vi "_goop4.llb_Interface_FindInterfaceImplementationVI.vi"(8 "error in (no error)":errorcluster, 10 "Path":path, 11 "LabVIEW Object in":refnum<class>) -> (0 "error out":errorcluster, 2 "VI Refnum Of Interface method in class":refnum<vi>, 3 "NoImplementationFound":bool, 5 "Full Class Name":string)   [LabVIEW 2014]
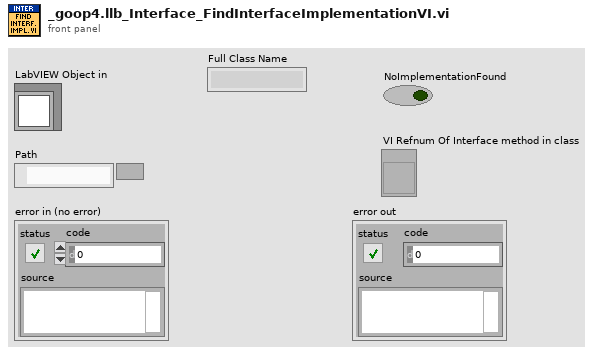
[diagram p1: front panel]
types:
  T1 = enum8{"Only include commented out diagrams if diagram already loaded", "Never include commented out diagrams", "Always include commented out diagrams"}
  T2 = enum8{"No dynamic dispatch VIs", "Include nearest implementation", "Include all overrides"}
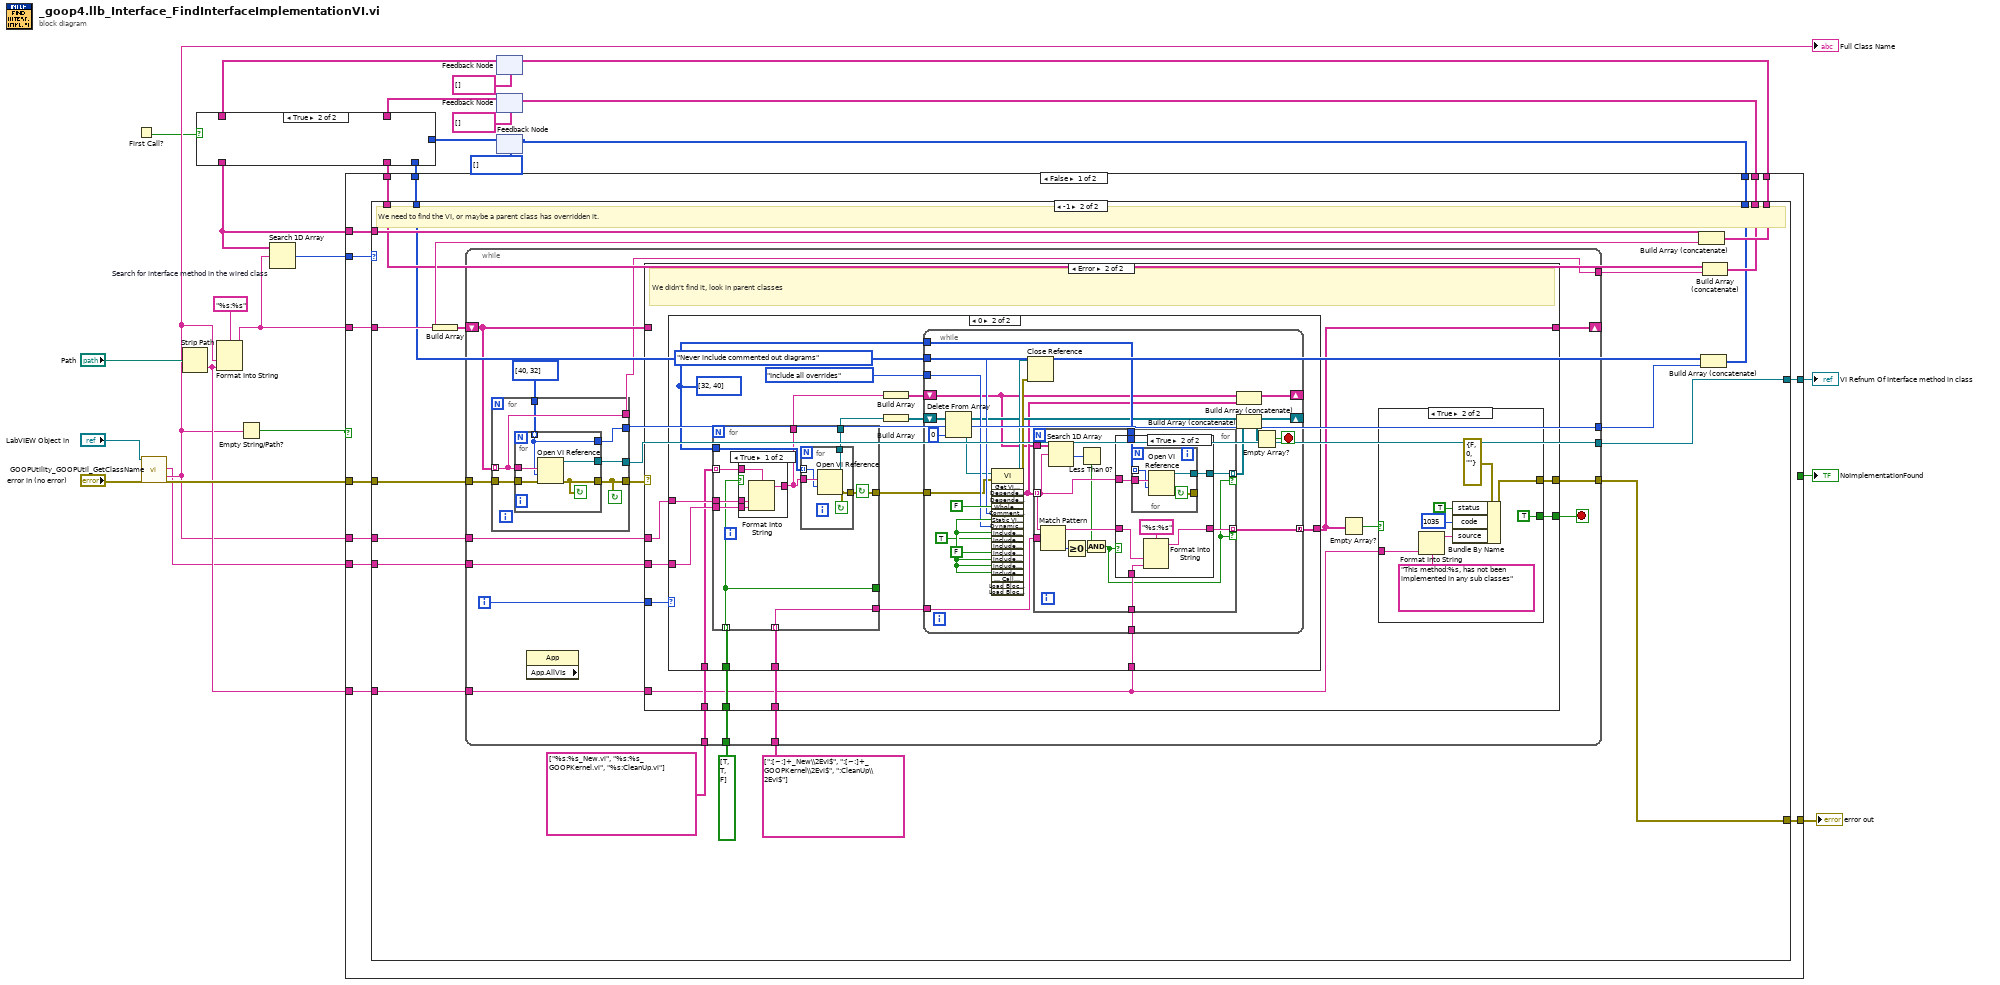
[diagram p0: block diagram]
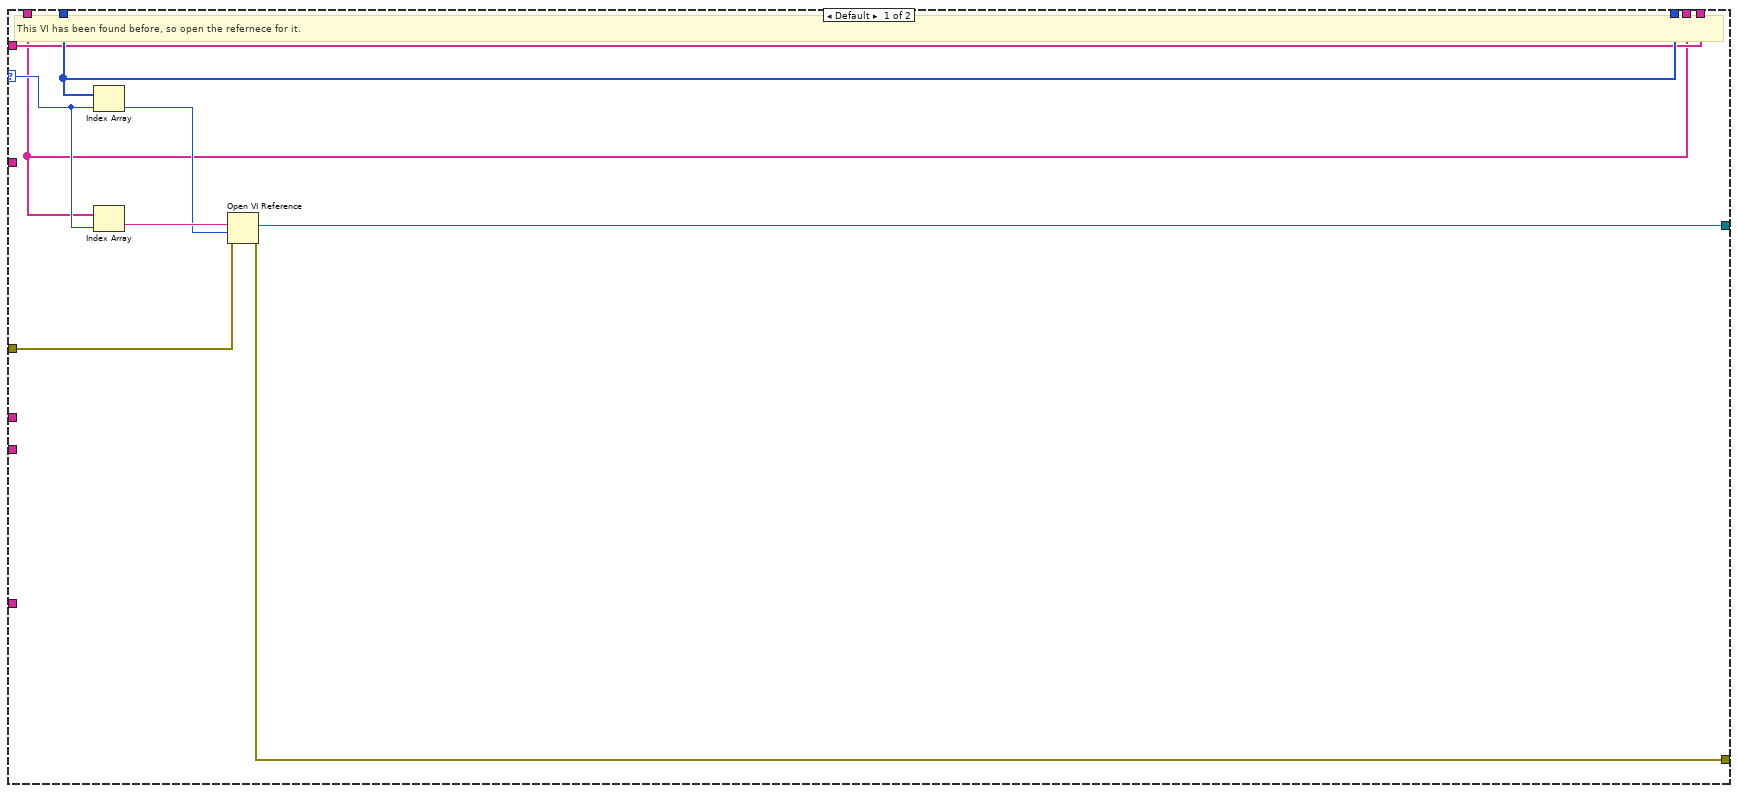
[diagram p2: hidden frame]
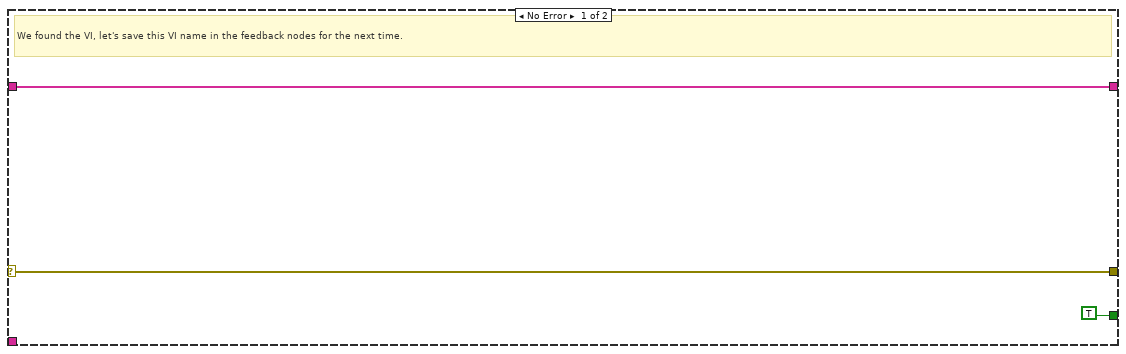
[diagram p3: hidden frame]
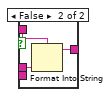
[diagram p6: hidden frame]
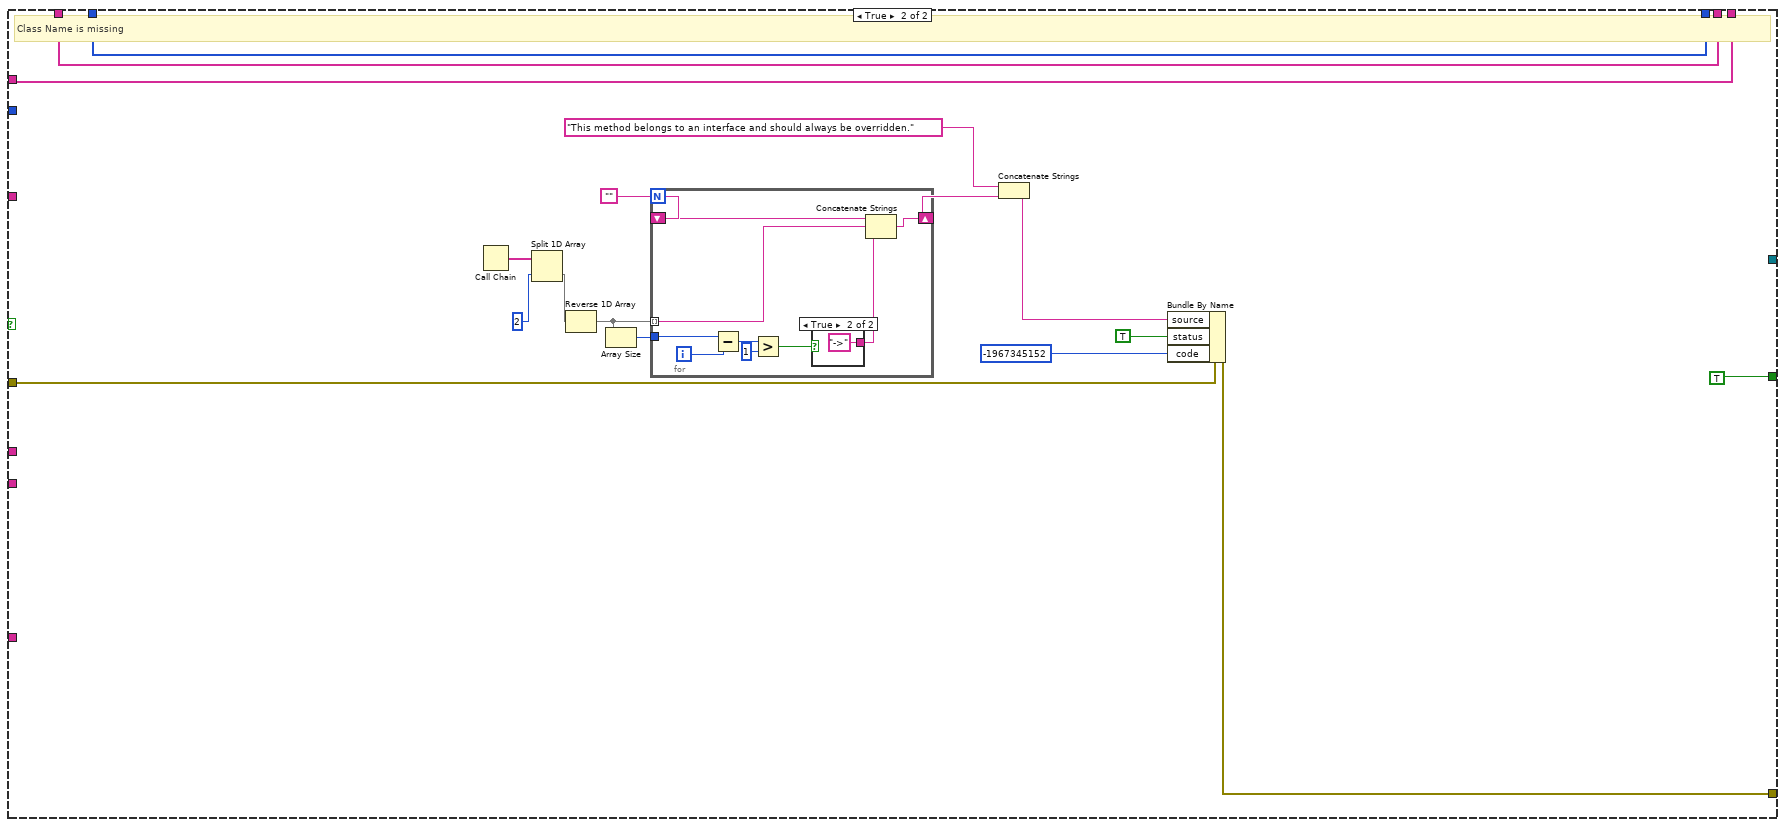
[diagram p8: hidden frame]
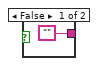
[diagram p9: hidden frame]
diagram:
  n1 = First Call?() -> (First Call?: T/F=w6:bool)
  n2 = call "GOOPUtility_GOOPUtil_GetClassName.vi"("LabVIEW Object"="LabVIEW Object in", "error in (no error)"="error in (no error)") -> ("Class Name"=w10:string, "Full Class Name"=w11:string, "error out"=w22:errorcluster)  [unwired: 13 in, 2 out]
  "Full Class Name" <- w11
  n3 = Strip Path(path="Path") -> (name=w12:string)  [unwired: 1 out]
  n4 = Format Into String(format string="%s:%s", w11, w12) -> (resulting string=w20:string)  [unwired: 2 in, 1 out]
  n5 = Empty String/Path?(string/path=w11) -> (empty?=w2:bool)
  n6 = feedback #1(string[] []) -> (w7:string[])
  n7 = feedback #2(string[] []) -> (w8:string[])
  n8 = feedback #3(i32[] []) -> (w9:i32[])
  n9 = case shown="True" w6 {
    tunnel: w9 -> [w28 _]
    tunnel: w8 -> [w29 _]
    tunnel: w7 -> [w30 _]
    tunnel: [w30 _] -> w5
    tunnel: [w29 _] -> w4
    tunnel: [w28 _] -> w3
    frame False {
    }
    frame True {
    }
  }
  n10 = Search 1D Array "Search for interface method in the wired class"(1D array=w5, element=w20) -> (index of element=w19:i32)  [unwired: 1 in]
  n11 = case shown="False" w2 {
    tunnel: [w44 _] -> w23
    tunnel: w22 -> [w43 w206]
    tunnel: [w42 w205] -> w21
    tunnel: w20 -> [w41 _]
    tunnel: w19 -> [w40 _]
    tunnel: [w39 w219] -> w16
    tunnel: [w38 w221] -> w15
    tunnel: [w37 w220] -> w13
    tunnel: w12 -> [w36 _]
    tunnel: w11 -> [w35 _]
    tunnel: w10 -> [w34 _]
    tunnel: w5 -> [w33 w221]
    tunnel: w4 -> [w32 w220]
    tunnel: w3 -> [w31 w219]
    tunnel: [_ TRUE] -> w1
    frame False {
      n12 = case shown="-1" w40 {
        selector: w40 -> [w51 _]
        tunnel: [w46 w72] -> w44
        tunnel: w43 -> [w48 w71]
        tunnel: [w47 w63] -> w42
        tunnel: w41 -> [_ w68]
        tunnel: w31 -> [w53 w65]
        tunnel: [w53 w64] -> w39
        tunnel: w33 -> [w52 w69]
        tunnel: [w52 w70] -> w38
        tunnel: w32 -> [w45 w67]
        tunnel: [w45 w66] -> w37
        tunnel: w36 -> [_ w62]
        tunnel: w35 -> [_ w58]
        tunnel: w34 -> [_ w57]
        frame Default {
          # "This VI has been found before, so open the refernece for it."
          n13 = Index Array(array=w53, index=w51) -> (element=w49:i32)
          n14 = Index Array(array=w45, index=w51) -> (element=w50:string)
          n15 = Open VI Reference(vi path=w50, options=w49, error in (no error)=w48) -> (vi reference=w46:refnum<vi>, error out=w47:errorcluster)  [unwired: 3 in]
        }
        frame -1 {
          # "We need to find the VI, or maybe a parent class has overridden it."
          n16 = Build Array(w68) -> (w61:string[])
          n17 = while {
            tunnel: [w82] -> w72
            tunnel: w71 -> [w89]
            shift-right: [w85] -> _
            shift-left: w61 -> [w86]
            tunnel: [w84] -> w63
            tunnel: w62 -> [w83]
            tunnel: [w81] -> w60
            tunnel: [w80] -> w59
            tunnel: w58 -> [w78]
            tunnel: w57 -> [w77]
            tunnel: bool[] [TRUE, TRUE, FALSE] -> [w76]
            tunnel: string[] ["%s:%s_New.vi", "%s:%s_GOOPKernel.vi", "%s:CleanUp.vi"] -> [w75]
            tunnel: string[] [":[~:]+_New\\2Evi$", ":[~:]+_GOOPKernel\\2Evi$", ":CleanUp\\2Evi$"] -> [w74]
            i -> [w79]
            stop <- w87 stop-if-true
            n18 = for {
              tunnel: i32[] [40, 32] -> [w91]
              tunnel: w89 -> [w95]
              tunnel: [w94] -> w88
              tunnel: [w93] -> w82
              tunnel: w86 -> [w92] mode=indexing
              tunnel: [w90] -> w81
              tunnel: [w92] -> w80
              stop <- w94 continue-if-true
              n19 = for {
                tunnel: w92 -> [w99]
                tunnel: [w98] -> w93
                tunnel: w91 -> [w96] mode=indexing
                tunnel: w95 -> [w100]
                tunnel: [w97] -> w94
                tunnel: [w96] -> w90
                stop <- w97 continue-if-true
                n20 = Open VI Reference(vi path=w99, options=w96, error in (no error)=w100) -> (vi reference=w98:refnum<vi>, error out=w97:errorcluster)  [unwired: 3 in]
              }
            }
            n21 = property class="App" props=["App.AllVIs"]() -> ()  [unwired: 2 in, 3 out]
            n22 = case shown="Error" w88 {
              selector: w88 -> [w101 _]
              tunnel: [TRUE w113] -> w87
              tunnel: w86 -> [w102 _]
              tunnel: [w102 w105] -> w85
              tunnel: [w101 w114] -> w84
              tunnel: w83 -> [_ w106]
              tunnel: w79 -> [_ w112]
              tunnel: w78 -> [_ w111]
              tunnel: w77 -> [_ w110]
              tunnel: w76 -> [_ w109]
              tunnel: w75 -> [_ w108]
              tunnel: w74 -> [_ w107]
              frame No Error {
                # "We found the VI, let's save this VI name in the feedback nodes for the next time."
              }
              frame Error {
                # "We didn't find it, look in parent classes"
                n23 = case shown="0" w112 {
                  tunnel: w111 -> [_ w130]
                  tunnel: w110 -> [_ w129]
                  tunnel: w109 -> [_ w128]
                  tunnel: w108 -> [_ w127]
                  tunnel: w107 -> [_ w126]
                  tunnel: w106 -> [_ w122]
                  tunnel: [_ w120] -> w105
                  frame Default {
                  }
                  frame 0 {
                    w115 = i32[] [32, 40]
                    n24 = for {
                      tunnel: [w181] -> w118
                      tunnel: [w180] -> w123
                      tunnel: w130 -> [w185]
                      tunnel: w127 -> [w184] mode=indexing
                      tunnel: w128 -> [w178] mode=indexing
                      tunnel: w129 -> [w183]
                      tunnel: [w182] -> w121
                      tunnel: w126 -> [w182] mode=indexing
                      tunnel: w115 -> [w179]
                      tunnel: [w178] -> _
                      tunnel: [w177] -> w116
                      stop <- w180 continue-if-true
                      n25 = case shown="True" w178 {
                        tunnel: [w193 w196] -> w177
                        tunnel: w185 -> [w192 w195]
                        tunnel: w184 -> [w191 w194]
                        tunnel: w183 -> [w190 _]
                        frame True {
                          n26 = Format Into String(format string=w191, w192, w190) -> (resulting string=w193:string)  [unwired: 2 in, 1 out]
                        }
                        frame False {
                          n27 = Format Into String(format string=w194, w195) -> (resulting string=w196:string)  [unwired: 2 in, 1 out]
                        }
                      }
                      n28 = for {
                        tunnel: w177 -> [w189]
                        tunnel: [w188] -> w181
                        tunnel: w179 -> [w187] mode=indexing
                        tunnel: [w186] -> w180
                        stop <- w186 continue-if-true
                        n29 = Open VI Reference(vi path=w189, options=w187) -> (vi reference=w188:refnum<vi>, error out=w186:errorcluster)  [unwired: 4 in]
                      }
                    }
                    n30 = Build Array(w116) -> (w117:string[])
                    n31 = Build Array(w118) -> (w119:refnum<vi>[])
                    n32 = while {
                      tunnel: T2."Include all overrides" ("Dynamic Dispatching?") -> [w143]
                      tunnel: T1."Never include commented out diagrams" ("Commented Out Diagrams?") -> [w144]
                      tunnel: w123 -> [w141]
                      tunnel: w122 -> [w148]
                      tunnel: w121 -> [w147]
                      tunnel: [w146] -> w120 mode=concatenating
                      shift-right: [w135] -> _
                      shift-left: w119 -> [w140]
                      tunnel: w115 -> [w138]
                      shift-right: [w131] -> _
                      shift-left: w117 -> [w132]
                      stop <- w134 stop-if-true
                      w152 = FALSE ("Include Poly VIs?")
                      n33 = Delete From Array(array=w140, index=0) -> (deleted portion=w142:refnum<vi>, array with subset deleted=w136:refnum<vi>[])  [unwired: 1 in]
                      n34 = invoke class="VI" method="Get VI Dependencies"(reference=w142, error in=w141, "Whole Hierarchy?"=FALSE, "Commented Out?"=w144, "Static VI Refs?"=w152, "Dynamic Dispatching?"=w143, "Include Missing VIs?"=w152, "Include Standard VIs?"=TRUE, "Include Poly VIs?"=w152, "Include Global VIs?"=w152, "Include Control VIs?"=w152, "Include Generic VIs?"=w152) -> (reference out=w149:refnum<vi>, error out=w150:errorcluster, "Dependency Names"=w133:string[])  [unwired: 7 in, 16 out]
                      n35 = Close Reference(reference=w149, error in (no error)=w150) -> ()  [unwired: 1 out]
                      n36 = for {
                        tunnel: w147 -> [w161]
                        tunnel: w133 -> [w157] mode=indexing
                        tunnel: [w162] -> w146 mode=indexing if=w153
                        tunnel: w148 -> [w163]
                        tunnel: w138 -> [w160]
                        tunnel: [w159] -> w137 mode=indexing if=w153
                        tunnel: w132 -> [w158]
                        n37 = Match Pattern(string=w157, regular expression=w161) -> (before substring=w164:string, offset past match=w165:i32)  [unwired: 1 in, 2 out]
                        n38 = Search 1D Array(1D array=w158, element=w157) -> (index of element=w156:i32)  [unwired: 1 in]
                        n39 = Greater Or Equal To 0?(x=w165) -> (x >= 0?=w155:bool)
                        n40 = Less Than 0?(x=w156) -> (x < 0?=w154:bool)
                        n41 = And(x=w154, y=w155) -> (x .and. y?=w153:bool)
                        n42 = case shown="True" w153 {
                          tunnel: w164 -> [_ w171]
                          tunnel: w163 -> [_ w170]
                          tunnel: [_ w169] -> w162
                          tunnel: w157 -> [_ w168]
                          tunnel: w160 -> [_ w167]
                          tunnel: [_ w166] -> w159
                          frame False {
                          }
                          frame True {
                            n43 = for {
                              tunnel: w168 -> [w176]
                              tunnel: [w175] -> w166
                              tunnel: w167 -> [w174] mode=indexing
                              tunnel: [w173] -> _
                              stop <- w173 continue-if-true
                              n44 = Open VI Reference(vi path=w176, options=w174) -> (vi reference=w175:refnum<vi>, error out=w173:errorcluster)  [unwired: 4 in]
                            }
                            n45 = Format Into String(format string="%s:%s", w171, w170) -> (resulting string=w169:string)  [unwired: 2 in, 1 out]
                          }
                        }
                      }
                      n46 = Build Array (concatenate)(w132, w133) -> (w131:string[])
                      n47 = Build Array (concatenate)(w136, w137) -> (w135:refnum<vi>[])
                      n48 = Empty Array?(array=w135) -> (empty?=w134:bool)
                    }
                  }
                }
                n49 = Empty Array?(array=w105) -> (empty?=w104:bool)
                n50 = case shown="True" w104 {
                  tunnel: [_ w204] -> w114
                  tunnel: [_ TRUE] -> w113
                  tunnel: w106 -> [_ w200]
                  frame False {
                  }
                  frame True {
                    n51 = Format Into String(format string="This method:%s, has not been implemented in any sub classes" ("string"), w200) -> (resulting string=w201:string)  [unwired: 2 in, 1 out]
                    n52 = Bundle By Name(cluster=errorcluster {"status"=FALSE, "code"=0, "source"=""} ("error IO"), "status"=TRUE, "code"=1035, "source"=w201) -> (w204:errorcluster)
                  }
                }
              }
            }
          }
          n53 = Build Array (concatenate)(w69, w68) -> (w70:string[])
          n54 = Build Array (concatenate)(w65, w60) -> (w64:i32[])
          n55 = Build Array (concatenate)(w67, w59) -> (w66:string[])
        }
      }
    }
    frame True {
      # "Class Name is missing"
      n56 = Call Chain() -> (call chain=w217:string[])
      n57 = Split 1D Array(array=w217, index=2) -> (second subarray=w215:string[])  [unwired: 1 out]
      n58 = Reverse 1D Array(array=w215) -> (reversed array=w212:string[])
      n59 = Array Size(array=w212) -> (size(s)=w214:i32)
      n60 = for {
        shift-right: [w222] -> w210
        shift-left: "" -> [w225]
        tunnel: w212 -> [w223] mode=indexing
        tunnel: w214 -> [w230]
        i -> [w229]
        n61 = Subtract(x=w230, y=w229) -> (x-y=w228:i32)
        n62 = Greater?(x=w228, y=1) -> (0:w226:bool)
        n63 = case shown="True" w226 {
          tunnel: ["" "->"] -> w224
          frame False {
          }
          frame True {
          }
        }
        n64 = Concatenate Strings(w225, w223, w224) -> (w222:string)
      }
      n65 = Concatenate Strings("This method belongs to an interface and should always be overridden." ("string"), w210) -> (w209:string)
      n66 = Bundle By Name(cluster=w206, "source"=w209, "status"=TRUE, "code"=-1967345152) -> (w205:errorcluster)
    }
  }
  "error out" <- w21
  "NoImplementationFound" <- w1
  "VI Refnum Of Interface method in class" <- w23
  n67 = feedback-in #1(w15) -> ()
  n68 = feedback-in #2(w13) -> ()
  n69 = feedback-in #3(w16) -> ()
